vi "analog_input.vi"(2 "save values?":bool, 4 "Voltage Log File Path":path=path "C:/data/Voltage Log Files/voltagelog11072007.txt", 5 "?":bool[](array[boolean])=[TRUE, TRUE, TRUE, TRUE, TRUE, TRUE, TRUE, TRUE, TRUE, TRUE, TRUE, TRUE, TRUE, TRUE, TRUE, TRUE], 6 "error in":errorcluster) -> (0 "error out":errorcluster, 1 "Data display":T1(graph), 3 "Array Out":dbl[](array[numeric])=[0.02140581164736354, 0.006151220255907583, 5.116805524879685, 0.0, 0.0, 0.0, 0.0, 0.0, 0.0, 0.0, 0.0, 0.0, 0.0, 0.0, 0.0, 0.0] format="%.6f")   [LabVIEW 2013]
uses:
  <vilib>/DAQmx/read.llb/DAQmx Read (Analog 1D DBL NChan 1Samp).vi
  <vilib>/DAQmx/miscellaneous.llb/DAQmx Fill In Error Info.vi
panel:
  out "Numeric":i32
  out "?":bool
  in  "stop":bool=TRUE
  # "Signal"
  # "Channel 1"
  # "Channel 2"
  # "Channel 3"
  # "Channel 4"
  # "Channel 5"
  # "Channel 6"
  # "Channel 7"
  # "Channel 8"
  # "Channel 9"
  # "Channel 10"
  # "Channel 11"
  # "Channel 12"
  # "Channel 13"
  # "Channel 14"
  # "Channel 15"
  # "Channel 16"
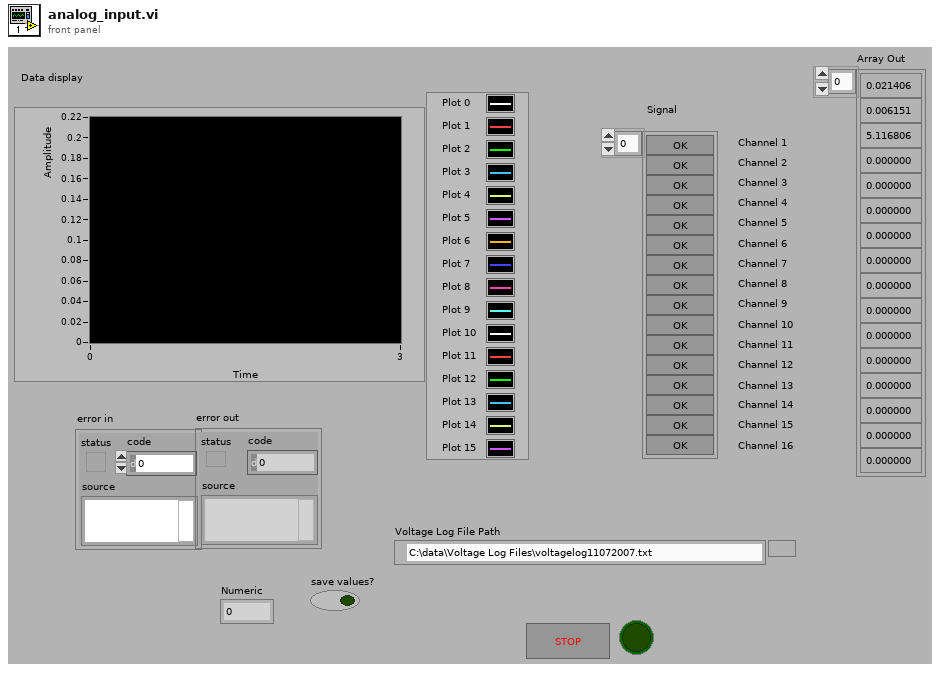
[diagram p1: front panel]
types:
  T1 = cluster{"data[0]":dbl, "data[1]":dbl, "data[2]":dbl, "data[3]":dbl, "data[4]":dbl, "data[5]":dbl, "data[6]":dbl, "data[7]":dbl, "data[8]":dbl, "data[9]":dbl, "data[10]":dbl, "data[11]":dbl, "data[12]":dbl, "data[13]":dbl, "data[14]":dbl, "data[15]":dbl}
  T2 = cluster{"Array Out 3[0]":dbl, "Array Out 3[1]":dbl, "Array Out 3[2]":dbl, "Array Out 3[3]":dbl, "Array Out 3[4]":dbl, "Array Out 3[5]":dbl, "Array Out 3[6]":dbl, "Array Out 3[7]":dbl, "Array Out 3[8]":dbl, "Array Out 3[9]":dbl, "Array Out 3[10]":dbl, "Array Out 3[11]":dbl, "Array Out 3[12]":dbl, "Array Out 3[13]":dbl, "Array Out 3[14]":dbl, "Array Out 3[15]":dbl}
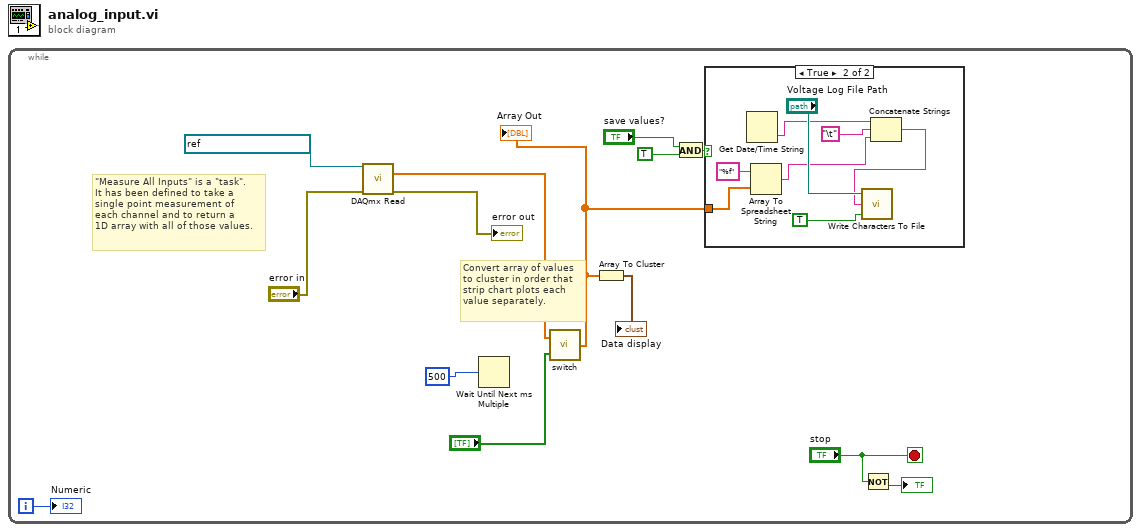
[diagram p0: block diagram]
diagram:
  n1 = while {
    i -> [w5]
    stop <- "stop" stop-if-true
    # "Convert array of values\nto cluster in order that\nstrip chart plots each\nvalue separately."
    # "\"Measure All Inputs\" is a \"task\".\nIt has been defined to take a\nsingle point measurement of\neach channel and to return a\n1D array with all of those values."
    n2 = call-poly <vilib>:"DAQmx Read.vi"("task/channels in"=refnum<k21> "Measure All Inputs", "error in"="error in") -> ("data"=w8:dbl[], "error out"=→"error out":errorcluster)  [unwired: 11 in, 1 out]
    n3 = Wait Until Next ms Multiple(millisecond multiple=u32 500 ("millisecond timer value")) -> ()  [unwired: 1 out]
    n4 = call "switch.vi"("Array 2"="?", "Array 4"=w8) -> ("Array Out 3"=w1:dbl[])
    "Array Out" <- w1
    n5 = Array To Cluster(array=w1) -> (cluster=→"Data display":T2)
    n6 = And(x="save values?", y=TRUE) -> (x .and. y?=w4:bool)
    n7 = case shown="True" w4 {
      tunnel: w1 -> [_ w17]
      frame False {
      }
      frame True {
        n8 = Get Date/Time String() -> (time string=w20:string)  [unwired: 3 in, 1 out]
        n9 = Array To Spreadsheet String(array=w17, 3:"%f" ("format string")) -> (spreadsheet string=w16:string)  [unwired: 1 in]
        n10 = Concatenate Strings(w20, "\t", w16) -> (w21:string)
        n11 = call <vilib>:"Write Characters To File.vi"("append to file? (new file:F)"=TRUE, "character string"=w21, "file path (dialog if empty)"="Voltage Log File Path") -> ()  [unwired: 2 in, 1 out]
      }
    }
    n12 = Not(x="stop") -> (.not. x?=→"?":bool)
    "Numeric" <- w5
  }
